vi "Iterpolate Data for NaN Array Values.vi"(10 "Y in":dbl[](array[numeric])=[0.9888395293291312, 0.3646147092585469, 2.0850251780938986, 2.6822138633389514, 1.868607599545117, 1.9237825677302502, 2.414110207699311, nan, 2.08801861471526, 3.64583177347688, 3.7315066551301292]) -> (2 "Y Repaiered":dbl[](array[numeric]))   [LabVIEW 2014]
doc: "This VI takes an Array with NaN (not a Number) values and iterpolates new values to fill in for the NaN data. \n\nThis VI designed to work with data with a constant delta X value. and this algorythm will not work for generating the first or last datapoint in an array."
panel:
  out "Y Data":cluster{i32[], "Y raw":dbl[]}[](graph)
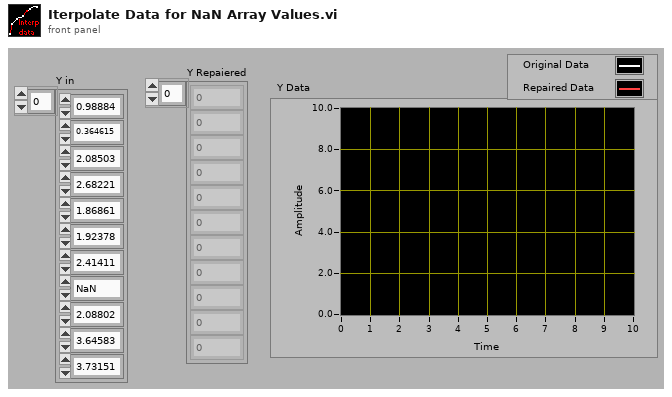
[diagram p1: front panel]
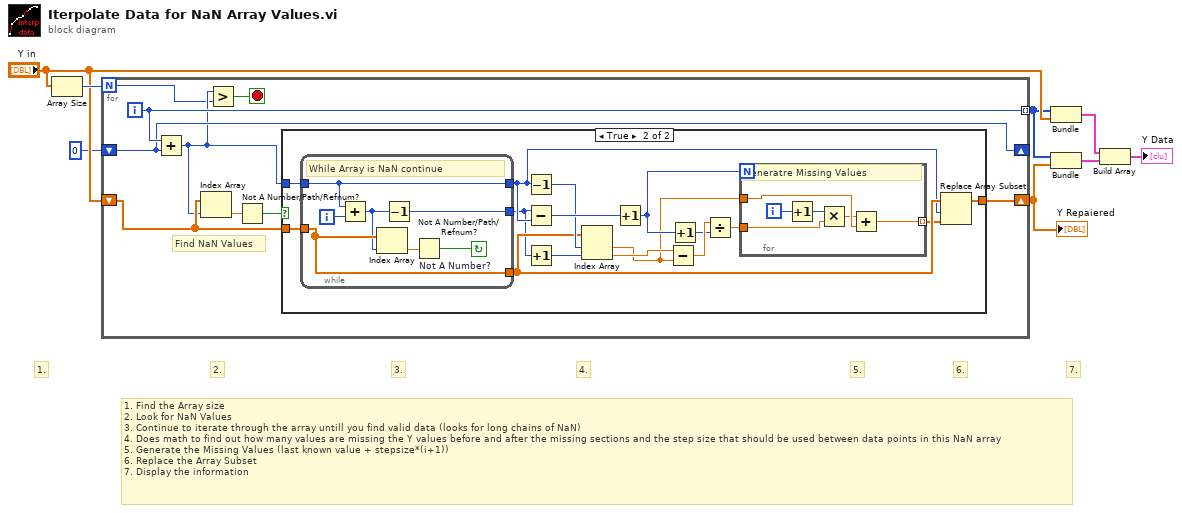
[diagram p0: block diagram]
diagram:
  # "1. Find the Array size\n2. Look for NaN Values\n3. Continue to iterate through the array untill you find valid data (looks for long chains of NaN)\n4. Does math to find out how many values are missing the Y values before and after the missing sections and the step size that should be used between data points in this NaN array\n5. Generate the Missing Values (last known value + stepsize*(i+1))\n6. Replace the Array Subset\n7. Display the information"
  # "7."
  # "6."
  # "5."
  # "4."
  # "3."
  # "2."
  # "1."
  n1 = Array Size(array="Y in") -> (size(s)=w8:i32)
  n2 = for {
    N: w8 -> [w10]
    shift-right: [w15] -> w7
    shift-left: "Y in" -> [w12]
    tunnel: [w14] -> w5 mode=indexing
    shift-right: [w13] -> _
    shift-left: 0 -> [w13]
    i -> [w14]
    stop <- w9 stop-if-true
    # "Find NaN Values"
    n3 = Add(x=w14, y=w13) -> (x+y=w11:i32)
    n4 = Index Array "Index Array"(array=w12, index=w11) -> (element=w17:dbl)
    n5 = Greater?(x=w11, y=w10) -> (0:w9:bool)
    n6 = Not A Number/Path/Refnum?(number/path/refnum=w17) -> (NaN/Path/Refnum?=w16:bool)
    n7 = case shown="True" w16 {
      tunnel: w11 -> [_ w34]
      tunnel: w12 -> [w18 w33]
      tunnel: [w18 w23] -> w15
      frame False {
      }
      frame True {
        n8 = while {
          tunnel: w34 -> [w47]
          tunnel: w33 -> [w45]
          tunnel: [w47] -> w24
          tunnel: [w44] -> w22
          tunnel: [w45] -> w26
          i -> [w46]
          stop <- w41 continue-if-true
          # "While Array is NaN continue"
          n9 = Add(x=w47, y=w46) -> (x+y=w43:i32)
          n10 = Index Array(array=w45, index=w43) -> (element=w42:dbl)
          n11 = Decrement(x=w43) -> (x-1=w44:i32)
          n12 = Not A Number/Path/Refnum? "Not A Number?"(number/path/refnum=w42) -> (NaN/Path/Refnum?=w41:bool)
        }
        n13 = Decrement(x=w24) -> (x-1=w31:i32)
        n14 = Subtract(x=w22, y=w24) -> (x-y=w32:i32)
        n15 = Increment(x=w22) -> (x+1=w21:i32)
        n16 = Index Array(array=w26, index #1=w31, index #2=w21) -> (element #1=w19:dbl, element #2=w20:dbl)
        n17 = Increment(x=w32) -> (x+1=w27:i32)
        n18 = Subtract(x=w20, y=w19) -> (x-y=w30:dbl)
        n19 = Increment(x=w27) -> (x+1=w29:i32)
        n20 = Divide(x=w30, y=w29) -> (x/y=w28:dbl)
        n21 = for {
          N: w27 -> [_]
          tunnel: w19 -> [w39]
          tunnel: w28 -> [w40]
          tunnel: [w37] -> w25 mode=indexing
          i -> [w36]
          # "Generatre Missing Values"
          n22 = Increment(x=w36) -> (x+1=w35:i32)
          n23 = Multiply(x=w35, y=w40) -> (x*y=w38:dbl)
          n24 = Add(x=w38, y=w39) -> (x+y=w37:dbl)
        }
        n25 = Replace Array Subset(array=w26, new element=w25, index=w24) -> (w23:dbl[])
      }
    }
  }
  "Y Repaiered" <- w7
  n26 = Bundle(w5, "Y in"="Y in") -> (w3:cluster{i32[], "Y in":dbl[]})  [unwired: 1 out]
  n27 = Bundle(w5, "Y in"=w7) -> (w4:cluster{i32[], "Y in":dbl[]})  [unwired: 1 out]
  n28 = Build Array(w3, w4) -> (→"Y Data":cluster{i32[], "Y in":dbl[]}[])
